vi "Test Boolean Event Type.vi"() -> ()   [LabVIEW 2021]
uses:
  Source/Event Bus/Support/Event Source/Polled_EventSource/Polled_EventSource.lvclass
  C:/Users/timst/Documents/Repositories/Omni-Bus/Source/Event Bus/Support/Event Source/Event_Source.lvclass
  Source/Event Bus/Support/Event Type/OnChange/Bool/OnChange_Boolean.lvclass
  C:/Users/timst/Documents/Repositories/Omni-Bus/Source/Event Bus/Support/Event_Polled Type.lvclass
  Source/Omni-Bus/Omni_Bus.lvclass
  Source/Local Bus/Support/Tag List Type.ctl
  <vilib>/Utility/Data Type/Type Definitions/Data Type.ctl
  Source/Local Bus/Local Bus.lvclass
  C:/Users/timst/Documents/Repositories/Omni-Bus/Source/Omni-Bus/Bus Access/Bus_Access.lvclass
  <vilib>/TSA/Abstract Data Classes/Abs_Types/Type/Abs_Type.lvclass/Abs_Type.ctl
  Source/Omni-Bus/Omni_Bus.lvclass/Omni_Bus.ctl
  Source/Event Bus/Support/Event Type/OnChange/Bool/OnChange_Boolean.lvclass/OnChange_Boolean.ctl
  Source/Event Bus/Support/Event Source/Event_Source.lvclass/Event_Source.ctl
  Source/Event Bus/Support/Event Source/Polled_EventSource/Polled_EventSource.lvclass/Polled_EventSource.ctl
  Source/Omni-Bus/Support/Get/Get Boolean.vi
  Source/Event Bus/Support/Event Type/OnChange/Bool/Properties/Write Data Type.vi
  Source/Event Bus/Support/Event Source/Properties/Write Events.vi
  Source/Event Bus/Support/Event Source/Polled_EventSource/Properties/Write Poll Interval (ms).vi
  Source/Omni-Bus/Support/FindVar.vi
  <vilib>/Utility/error.llb/Clear Errors.vi
  Source/Omni-Bus/Properties/Read Var Map.vi
  <vilib>/TSA/Abstract Data Classes/Abs_Types/Type/Properties/Read Tag.vi
  <vilib>/TSA/Abstract Data Classes/Abs_Types/Boolean/Abs_Boolean.lvclass
  C:/Program Files (x86)/National Instruments/LabVIEW 2021/vi.lib/TSA/Abstract Data Classes/Abs_Types/Type/Abs_Type.lvclass
  <vilib>/TSA/Abstract Data Classes/Abs_Types/Value/Abs_Value.lvclass
  Source/Omni-Bus/Support/Check For Read Only Error.vi
  Source/Omni-Bus/Support/Incorrect Tag String Error.vi
  <vilib>/TSA/Abstract Data Classes/Abs_Types/Type/Abs_Type.lvclass
  <vilib>/Utility/Data Type/NI_Data Type.lvlib
  C:/Users/timst/Documents/Repositories/Omni-Bus/Source/Local Bus/Local Bus.lvclass
  C:/Program Files (x86)/National Instruments/LabVIEW 2021/vi.lib/TSA/Abstract Data Classes/Abs_Types/Boolean/Abs_Boolean.lvclass
  C:/Program Files (x86)/National Instruments/LabVIEW 2021/vi.lib/TSA/Abstract Data Classes/Abs_Types/Value/Abs_Value.lvclass
  C:/Users/timst/Documents/Repositories/Omni-Bus/Source/Event Bus/Support/Event Type/Event_Type.lvclass
  C:/Users/timst/Documents/Repositories/Omni-Bus/Source/Event Bus/Support/Event Type/OnChange/Bool/OnChange_Boolean.lvclass
panel:
  out "Boolean 2":bool
  out "Numeric 2":i32
  in  "Boolean":bool
  out "Timeout":bool
  in  "stop 2":bool
  in  "stop":bool
  out "Numeric":i32
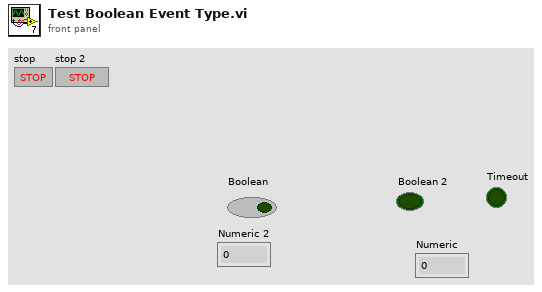
[diagram p1: front panel]
types:
  T1 = typedef "Local Bus.lvclass/Tag List Type.ctl" = cluster{"Tag":string, "Type":T2}
  T2 = typedef "NI_Data Type.lvlib/Data Type.ctl" = enum8{"Invalid Type", "Void", "I8", "I16", "I32", "I64", "U8", "U16", "U32", "U64", "Single Float", "Double Float", "Extended Float", "Single Complex", "Double Complex", "Extended Complex", "Enum U8", "Enum U16", "Enum U32", "Enum U64", "Single Float With Unit", "Double Float With Unit", "Extended Float With Unit", "Single Complex with Unit", "Double Complex with Unit", "Extended Complex with Unit", "Boolean", "String", "Path", "Picture", "Tag", "Array", "Cluster", "Variant", "LV Variant", "Waveform", "Timestamp", "Digital Waveform", "Digital Data", "ExpressData", "Refnum", "External Data", "VI", "Poly VI", "LabVIEW Class Instance", "Fixed Point", "Set Collection", "Map Collection"}
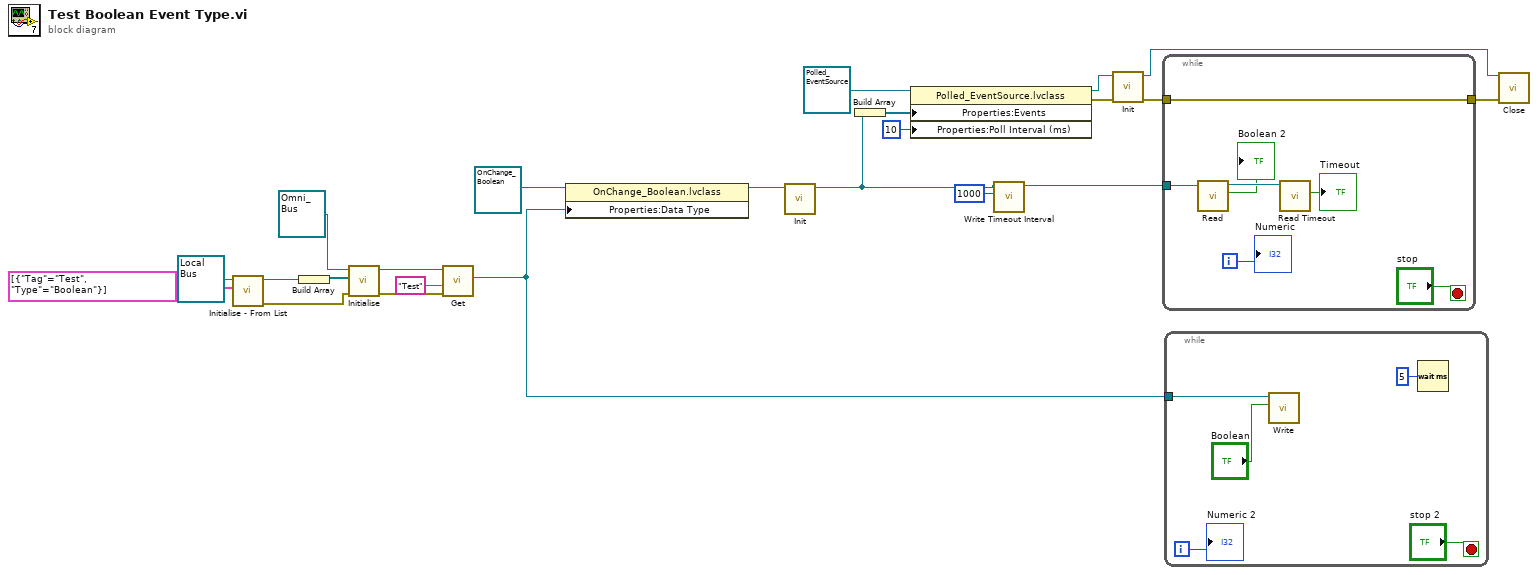
[diagram p0: block diagram]
diagram:
  n1 = call "Initialise - From List.vi"("Tag List"=T1[] [{"Tag"="Test", "Type"=enum."Boolean"}], "Local Bus in"=refnum<class "Local Bus.lvclass"> refnum) -> ("error out"=w15:errorcluster, "Local Bus out"=w17:refnum<class "Local Bus.lvclass">)  [unwired: 8 in]
  n2 = Build Array(w17) -> (w18:refnum<class "Local Bus.lvclass">[])
  n3 = call-dynamic "Initialise.vi"("error in (no error)"=w15, "Bus Access"=w18, "Var Bus in"=refnum<class "Omni_Bus.lvclass"> refnum) -> ("error out"=w20:errorcluster, "Var Bus out"=w21:refnum<class "Omni_Bus.lvclass">)  [unwired: 7 in]
  n4 = call-poly "Get.vi"("error in (no error)"=w20, "Tag"="Test", "Var Bus in"=w21) -> ("Value Out"=w8:refnum<class "Abs_Boolean.lvclass">)  [unwired: 5 in, 3 out]
  n5 = property class="OnChange_Boolean.lvclass"(reference=refnum<class "OnChange_Boolean.lvclass"> refnum ("OnChange_Boolean.lvclass"), "Properties:Data Type"=w8) -> (reference out=w2:refnum<class "OnChange_Boolean.lvclass">)  [unwired: 1 in, 1 out]
  n6 = call-dynamic "Init.vi"("Data in"=w2) -> ("Data out"=w1:refnum<class "OnChange_Boolean.lvclass">)  [unwired: 9 in, 1 out]
  n7 = Build Array(w1) -> (w14:refnum<class "OnChange_Boolean.lvclass">[])
  n8 = property class="Polled_EventSource.lvclass"(reference=refnum<class "Polled_EventSource.lvclass"> refnum ("Polled_EventSource.lvclass"), "Properties:Events"=w14, "Properties:Poll Interval (ms)"=10 ("Poll Interval (ms)")) -> (reference out=w12:refnum<class "Polled_EventSource.lvclass">, error out=w13:errorcluster)  [unwired: 1 in]
  n9 = call-dynamic "Write Timeout Interval.vi"("Timeout Interval (ms)"=1000, "OnChange_Boolean in"=w1) -> ("OnChange_Boolean out"=w7:refnum<class "OnChange_Boolean.lvclass">)  [unwired: 8 in, 1 out]
  n10 = call-dynamic "Init.vi"("error in (no error)"=w13, "Data in"=w12) -> ("error out"=w11:errorcluster, "Data out"=w9:refnum<class "Polled_EventSource.lvclass">)  [unwired: 8 in]
  n11 = while {
    tunnel: w7 -> [w27]
    tunnel: w11 -> [w28]
    tunnel: [w28] -> w10
    i -> [w30]
    stop <- "stop" stop-if-true
    n12 = call-dynamic "Read.vi"("Boolean in"=w27) -> ("Boolean"=→"Boolean 2":bool, "Boolean out"=w26:refnum<class "OnChange_Boolean.lvclass">)  [unwired: 8 in, 1 out]
    n13 = call-dynamic "Read Timeout.vi"("OnChange_Boolean in"=w26) -> ("Timeout"=→"Timeout":bool)  [unwired: 8 in, 2 out]
    "Numeric" <- w30
  }
  n14 = while {
    tunnel: w8 -> [w35]
    i -> [w31]
    stop <- "stop 2" stop-if-true
    n15 = call-dynamic "Write.vi"("Boolean"="Boolean", "Boolean in"=w35) -> ()  [unwired: 8 in, 2 out]
    n16 = Wait (ms)(milliseconds to wait=u32 5) -> ()  [unwired: 1 out]
    "Numeric 2" <- w31
  }
  n17 = call-dynamic "Close.vi"("error in (no error)"=w10, "Data in"=w9) -> ()  [unwired: 8 in, 2 out]
